vi "Sample_Panel_2.vi"(0 "HSMO#1":refnum<class "Hyper_State_Machine.lvclass">, 1 "State_Interval_Time(s)":dbl=0.025 min=0.0 max=86400.0 format="%#_13p", 2 "Time Target (s)":dbl=30.0 format="%#_13g", 3 "System_Delay(s)":dbl=0.05 min=0.0 max=86400.0 format="%#_13p") -> (8 "error out":errorcluster)   [LabVIEW 2021]
uses:
  C:/Program Files (x86)/Hyper State Machine Framework/SSW_Hyper_State_Machine.lvlibp/State_Machine_Class/Main_State_Machine/Hyper_State_Machine.lvclass
  C:/Program Files (x86)/Hyper State Machine Framework/SSW_Hyper_State_Machine.lvlibp/State_Machine_Class/State_Machine_Module.llb/State Machine.ctl
  C:/Program Files (x86)/Hyper State Machine Framework/SSW_Hyper_State_Machine.lvlibp/State_Machine_Class/State_Machine_Module.llb/State Machine[].ctl
  C:/Program Files (x86)/Hyper State Machine Framework/SSW_Hyper_State_Machine.lvlibp/State_Machine_Class/State_Machine_Module.llb/Iterval.ctl
  C:/Program Files (x86)/Hyper State Machine Framework/SSW_Hyper_State_Machine.lvlibp/State_Machine_Class/State_Machine_Module.llb/Lock_Unlock.ctl
  C:/Program Files (x86)/Hyper State Machine Framework/SSW_Hyper_State_Machine.lvlibp
panel:
  out "Running Mode":string
  out "This_State_Id":u32 format="%08x"
  out "Message from Child":string
  in  "Block Chain":bool=TRUE caption="Checkbox"
  in  "Message to Parent":string="I'm Child State"
  in  "Send":bool
  out "Parent_State_Id":u32 format="%08x"
  out "Panel_Close":bool=TRUE
  out "Active":bool=TRUE
  out "Implementation Class":string
  out "Current State":string
  out "Heartbeat":bool=TRUE
  in  "Unlock":bool
  in  "Reset":bool
  in  "lock All":bool
  in  "New_Windows":bool
  out "Timing":dbl
  out "Lock":bool
  # "HSMO#2"
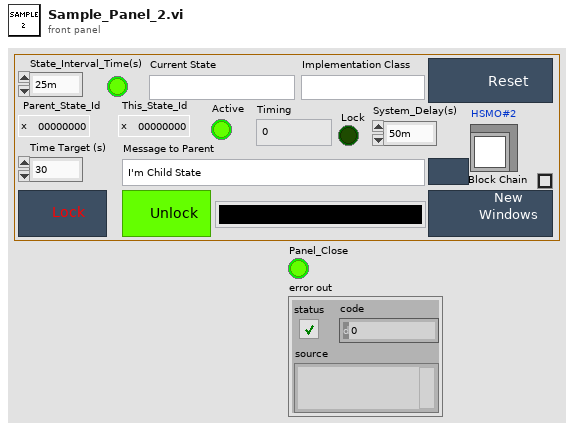
[diagram p1: front panel]
types:
  T1 = typedef "SSW_Hyper_State_Machine.lvlibp/State Machine.ctl" = cluster{"Command":string, "Data":variant}
  T2 = typedef "SSW_Hyper_State_Machine.lvlibp/Lock_Unlock.ctl" = cluster{"Action_Mode (Get)":enum16{"Set", "Get"}, "Action_Set (False)":bool, "State_In (Wait)":string}
  T3 = typedef "SSW_Hyper_State_Machine.lvlibp/State Machine[].ctl" = cluster{"Command":string, "Data":variant}[]
  T4 = typedef "SSW_Hyper_State_Machine.lvlibp/Iterval.ctl" = cluster{"Delay(s)":dbl, "State (Interval_Delay)":string}
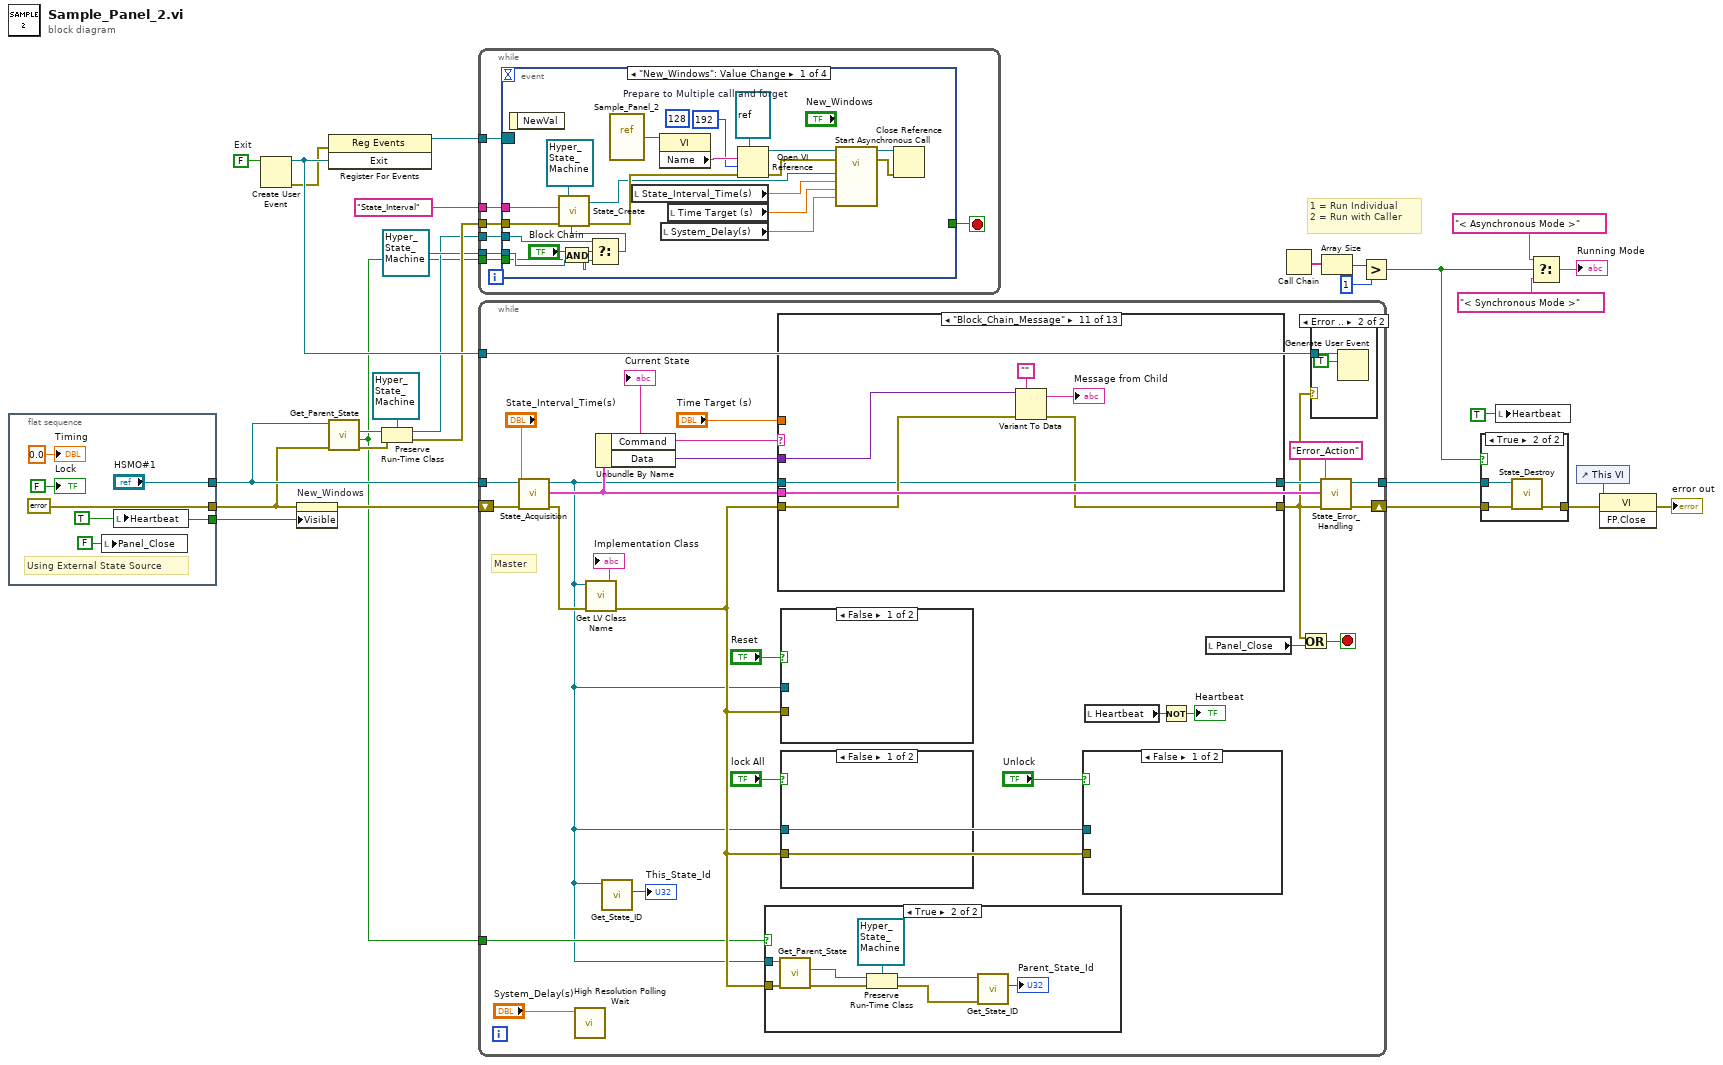
[diagram p0: block diagram]
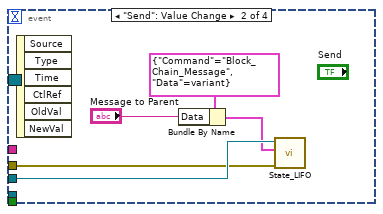
[diagram p3: hidden frame]
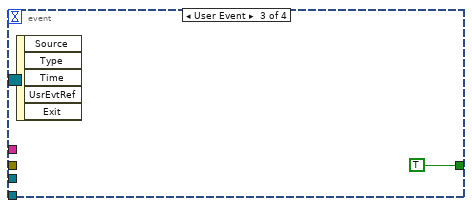
[diagram p4: hidden frame]
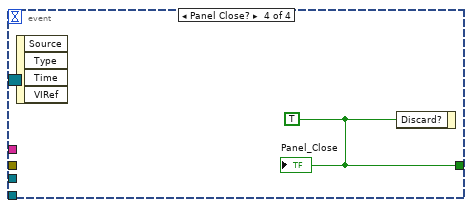
[diagram p5: hidden frame]
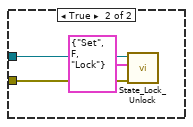
[diagram p8: hidden frame]
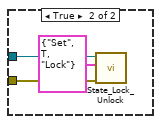
[diagram p9: hidden frame]
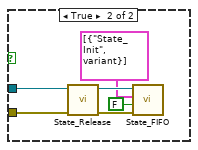
[diagram p10: hidden frame]
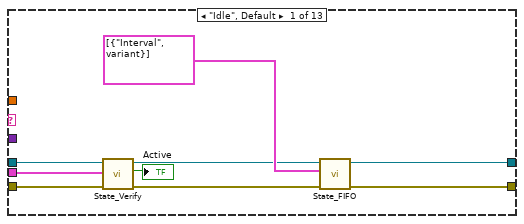
[diagram p11: hidden frame]
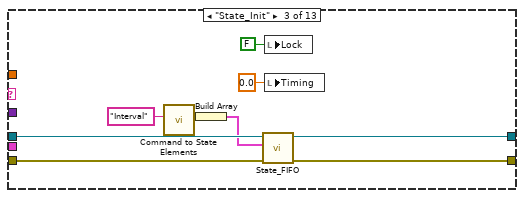
[diagram p13: hidden frame]
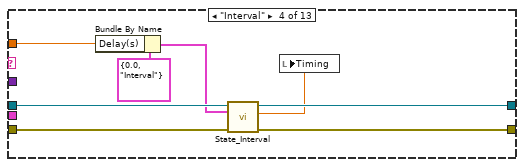
[diagram p14: hidden frame]
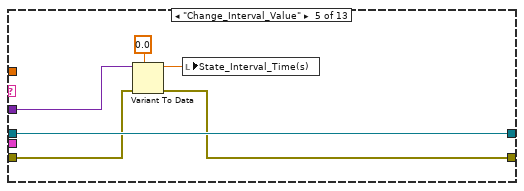
[diagram p15: hidden frame]
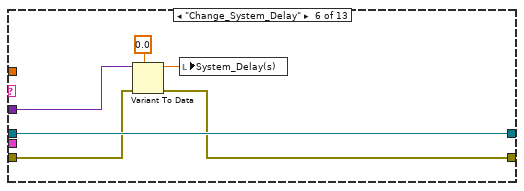
[diagram p16: hidden frame]
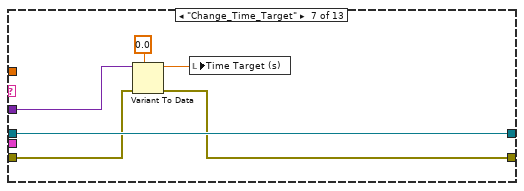
[diagram p17: hidden frame]
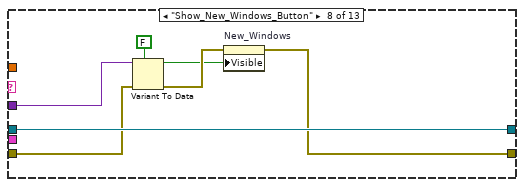
[diagram p18: hidden frame]
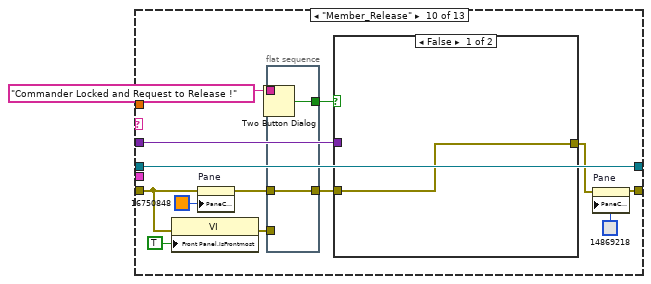
[diagram p20: hidden frame]
diagram:
  w26 = FALSE  # Exit
  # "1 = Run Individual\n2 = Run with Caller"
  n1 = flat-sequence {
    tunnel: ["HSMO#1"] -> w12
    tunnel: [errorcluster {"status"=FALSE, "code"=0, "source"=""} ("error out")] -> w11
    tunnel: [w31] -> w27
    frame #0 {
      w31 = TRUE ("Heartbeat")
      # "Using External State Source"
      n2 = local write "Panel_Close"(FALSE ("Panel_Close")) -> ()
      n3 = local write "Heartbeat"(w31) -> ()
      "Lock" <- FALSE ("Lock")
      "Timing" <- 0.0 ("Timing")
    }
  }
  n4 = Create User Event(user event datatype=w26) -> (user event=w24:refnum<user-event>, error out=w18:errorcluster)  [unwired: 1 in]
  n5 = property on="New_Windows" class="Bool"(error in=w11, "Visible"=w27) -> (error out=w28:errorcluster)  [unwired: 1 in, 1 out]
  n6 = register-events(error in=w18, w24) -> (reference out=w25:refnum<event-registration>)  [unwired: 1 in, 1 out]
  n7 = call-dynamic "Get_Parent_State.vi"("error in (no error)"=w11, "Hyper_State_Machine in"=w12) -> ("error out"=w10:errorcluster, "Paent_State_Status"=w9:bool, "Paent_State"=w13:refnum<class "State_Interface.lvclass">)  [unwired: 6 in, 1 out]
  n8 = Preserve Run-Time Class(object in=w13, error in=w10, 2:refnum<class "Hyper_State_Machine.lvclass"> refnum ("HSMO#1")) -> (object out=w14:refnum<class "Hyper_State_Machine.lvclass">, error out=w16:errorcluster)
  n9 = while {
    tunnel: w25 -> [w41]
    tunnel: "State_Interval" ("State_Interval_Name") -> [w40]
    tunnel: w16 -> [w39]
    tunnel: w14 -> [w38]
    tunnel: refnum<class "Hyper_State_Machine.lvclass"> refnum ("f") -> [w37]
    tunnel: w9 -> [w36]
    stop <- w42 stop-if-true
    n10 = event shown="[0] \"New_Windows\": Value Change" {
      selector: w41 -> [_ _ _ _]
      dyn-events: _ -> [_ _ _ _]
      timeout: _ -> [_ _ _ _]
      tunnel: [_ _ TRUE w71] -> w42
      tunnel: w40 -> [w52 _ _ _]
      tunnel: w39 -> [w51 w68 _ _]
      tunnel: w38 -> [w49 w69 _ _]
      tunnel: w37 -> [w48 _ _ _]
      tunnel: w36 -> [w44 _ _ _]
      event "New_Windows": Value Change {
        (unwired) 128 ("options")
        w43 = 192  # Prepare to Multiple call and forget
        n11 = event-data() -> ()  [unwired: 1 in, 1 out]
        n12 = And(x="Block Chain", y=w44) -> (x .and. y?=w45:bool)
        n13 = Select(t=w49, s=w45, f=w48) -> (s? t:f=w46:refnum<class "Hyper_State_Machine.lvclass">)
        n14 = call-dynamic "State_Create.vi"("Parent_State"=w46, "error in (no error)"=w51, "State_Interval_Name"=w52, "State_Machine_Class in"=refnum<class "Hyper_State_Machine.lvclass"> refnum) -> ("error out"=w53:errorcluster, "State_Machine_Class out"=w50:refnum<class "Hyper_State_Machine.lvclass">)  [unwired: 5 in, 1 out]
        n15 = vi-ref "Sample_Panel_2.vi"() -> (w64:refnum<vi>)
        n16 = local read "State_Interval_Time(s)"() -> (w57:dbl)
        n17 = property class="VI"(reference=w64) -> ("Name"=w63:string)  [unwired: 1 in, 2 out]
        n18 = local read "System_Delay(s)"() -> (w55:dbl)
        n19 = local read "Time Target (s)"() -> (w56:dbl)
        n20 = Open VI Reference(type specifier VI Refnum (for type only)=refnum<vi> refnum, vi path=w63, options=w43, error in (no error)=w53) -> (vi reference=w61:refnum<vi>, error out=w60:errorcluster)  [unwired: 2 in]
        n21 = call-by-ref "Start Asynchronous Call"(reference=w61, error in=w60, "HSMO#1"=w50, "State_Interval_Time(s)"=w57, "Time Target (s)"=w56, "System_Delay(s)"=w55) -> (reference out=w59:refnum<vi>, error out=w58:errorcluster)  [unwired: 4 in, 1 out]
        n22 = Close Reference(reference=w59, error in (no error)=w58) -> ()  [unwired: 1 out]
      }
      event "Send": Value Change {
        n23 = event-data() -> ()  [unwired: 1 in, 6 out]
        n24 = Bundle By Name(cluster=T1 {"Command"="Block_Chain_Message", "Data"=variant} ("State Machine"), "Data"="Message to Parent") -> (w65:T1)
        n25 = call-dynamic "State_LIFO.vi"("error in (no error)"=w68, "State Machine"=w65, "State_Machine_Class in"=w69) -> ()  [unwired: 7 in, 2 out]
      }
      event User Event {
        n26 = event-data() -> ()  [unwired: 1 in, 5 out]
      }
      event Panel Close? {
        w71 = TRUE ("Discard?")
        n27 = event-data() -> ()  [unwired: 1 in, 4 out]
        n28 = event-data("Discard?"=w71) -> ()  [unwired: 1 in, 1 out]
        "Panel_Close" <- w71
      }
    }
  }
  n29 = while {
    tunnel: w12 -> [w98]
    shift-right: [w80] -> w29
    shift-left: w28 -> [w97]
    tunnel: w24 -> [w81]
    tunnel: [w79] -> w20
    tunnel: w9 -> [w74]
    stop <- w76 stop-if-true
    # "Master"
    n30 = call-dynamic "State_Acquisition.vi"("error in (no error)"=w97, "State_Interval_Time(s)"="State_Interval_Time(s)", "Main_Machine_State_Class in"=w98) -> ("error out"=w84:errorcluster, "State"=w82:T1, "Main_Machine_State_Class out"=w72:refnum<class "Hyper_State_Machine.lvclass">)  [unwired: 2 in, 4 out]
    n31 = call <vilib>:"High Resolution Polling Wait.vi"("seconds to wait"="System_Delay(s)") -> ()  [unwired: 10 in, 1 out]
    n32 = call <vilib>:"Get LV Class Name.vi"("error in (no error)"=w84, "object"=w72) -> ("error out"=w75:errorcluster, "class name"=→"Implementation Class":string)  [unwired: 8 in]
    n33 = Unbundle By Name(w82) -> ("Command"=w86:string, "Data"=w89:variant)
    "Current State" <- w86
    n34 = call-dynamic "Get_State_ID.vi"("Hyper_State_Machine in"=w72) -> ("State_ID"=→"This_State_Id":u32)  [unwired: 8 in, 2 out]
    n35 = case shown="True" w74 {
      tunnel: w72 -> [_ w102]
      tunnel: w75 -> [_ w101]
      frame False {
      }
      frame True {
        n36 = call-dynamic "Get_Parent_State.vi"("error in (no error)"=w101, "Hyper_State_Machine in"=w102) -> ("error out"=w99:errorcluster, "Paent_State"=w100:refnum<class "State_Interface.lvclass">)  [unwired: 6 in, 2 out]
        n37 = Preserve Run-Time Class(object in=w100, error in=w99, 2:refnum<class "Hyper_State_Machine.lvclass"> refnum ("HSMO#1")) -> (object out=w104:refnum<class "Hyper_State_Machine.lvclass">, error out=w103:errorcluster)
        n38 = call-dynamic "Get_State_ID.vi"("error in (no error)"=w103, "Hyper_State_Machine in"=w104) -> ("State_ID"=→"Parent_State_Id":u32)  [unwired: 7 in, 2 out]
      }
    }
    n39 = case shown="\"Block_Chain_Message\"" w86 {
      tunnel: w89 -> [_ _ _ _ w153 w159 w165 w172 _ w187 w204 _ _]
      tunnel: w72 -> [w126 w131 w140 w146 w154 w160 w166 w173 w175 w188 w202 w211 w218]
      tunnel: w75 -> [w125 w130 w138 w145 w152 w158 w164 w171 w174 w182 w203 w210 w217]
      tunnel: [w129 w131 w139 w143 w154 w160 w166 w173 w175 w188 w202 w209 w216] -> w87
      tunnel: [w128 w130 w137 w142 w151 w157 w163 w167 w174 w177 w201 w208 w212] -> w77
      tunnel: "Time Target (s)" -> [_ _ _ w148 _ _ _ _ _ _ _ _ _]
      tunnel: w82 -> [w124 _ _ _ _ _ _ _ _ _ _ _ _]
      frame "Idle", Default {
        n40 = call-dynamic "State_Verify.vi"("error in (no error)"=w125, "State(Idle)"=w124, "State_Machine_Class in"=w126) -> ("error out"=w122:errorcluster, "Active"=→"Active":bool, "State_Machine_Class out"=w123:refnum<class "Hyper_State_Machine.lvclass">)  [unwired: 6 in]
        n41 = call-dynamic "State_FIFO.vi"("error in (no error)"=w122, "State Machine[]"=T3 [{"Command"="Interval", "Data"=variant}], "State_Machine_Class in"=w123) -> ("error out"=w128:errorcluster, "State_Machine_Class out"=w129:refnum<class "Hyper_State_Machine.lvclass">)  [unwired: 7 in]
      }
      frame "State_Interval" {
        # "Execute Every Define of State Interval Time"
      }
      frame "State_Init" {
        n42 = call "Command to State Elements.vi"("Command"="Interval") -> ("Command to State Elements"=w135:T1)  [unwired: 10 in]
        n43 = Build Array(w135) -> (w134:T1[])
        n44 = call-dynamic "State_FIFO.vi"("error in (no error)"=w138, "State Machine[]"=w134, "State_Machine_Class in"=w140) -> ("error out"=w137:errorcluster, "State_Machine_Class out"=w139:refnum<class "Hyper_State_Machine.lvclass">)  [unwired: 7 in]
        n45 = local write "Lock"(FALSE ("Lock")) -> ()
        n46 = local write "Timing"(0.0 ("Timing")) -> ()
      }
      frame "Interval" {
        n47 = Bundle By Name(cluster=T4 {"Delay(s)"=0.0, "State (Interval_Delay)"="Interval"} ("Parameter"), "Delay(s)"=w148) -> (w144:T4)
        n48 = call-dynamic "State_Interval.vi"("error in (no error)"=w145, "Parameter"=w144, "State_Machine_Class in"=w146) -> ("error out"=w142:errorcluster, "Elapsed Time(s)"=w141:dbl, "State_Machine_Class out"=w143:refnum<class "Hyper_State_Machine.lvclass">)  [unwired: 6 in]
        n49 = local write "Timing"(w141) -> ()
      }
      frame "Change_Interval_Value" {
        n50 = Variant To Data(error in=w152, type=0.0 ("Time Target (s)"), Variant=w153) -> (data=w149:dbl, error out=w151:errorcluster)
        n51 = local write "State_Interval_Time(s)"(w149) -> ()
      }
      frame "Change_System_Delay" {
        n52 = Variant To Data(error in=w158, type=0.0 ("Time Target (s)"), Variant=w159) -> (data=w155:dbl, error out=w157:errorcluster)
        n53 = local write "System_Delay(s)"(w155) -> ()
      }
      frame "Change_Time_Target" {
        n54 = Variant To Data(error in=w164, type=0.0 ("Time Target (s)"), Variant=w165) -> (data=w161:dbl, error out=w163:errorcluster)
        n55 = local write "Time Target (s)"(w161) -> ()
      }
      frame "Show_New_Windows_Button" {
        n56 = Variant To Data(error in=w171, type=FALSE, Variant=w172) -> (data=w168:bool, error out=w169:errorcluster)
        n57 = property on="New_Windows" class="Bool"(error in=w169, "Visible"=w168) -> (error out=w167:errorcluster)  [unwired: 1 in, 1 out]
      }
      frame "Error_Action" {
      }
      frame "Member_Release" {
        n58 = property class="VI"(error in=w182, "Front Panel.IsFrontmost"=TRUE ("Front Panel Window:Is Frontmost")) -> (error out=w176:errorcluster)  [unwired: 1 in, 1 out]
        n59 = property on="Pane" class="Pane"(error in=w182, "PaneColor"=u32 16750848 ("Pane Color")) -> (error out=w181:errorcluster)  [unwired: 1 in, 1 out]
        n60 = flat-sequence {
          tunnel: "Commander Locked and Request to Release !" ("message") -> [w191]
          tunnel: [w190] -> w185
          tunnel: [w189] -> w180
          tunnel: w181 -> [w189]
          tunnel: w176 -> [_]
          frame #0 {
            n61 = Two Button Dialog(message=w191) -> (T button?=w190:bool)  [unwired: 2 in]
          }
        }
        n62 = case shown="False" w185 {
          tunnel: w180 -> [w192 w199]
          tunnel: w187 -> [_ w198]
          tunnel: [w192 w197] -> w178
          frame False {
          }
          frame True {
            n63 = Variant To Data(error in=w199, type=refnum<class "Hyper_State_Machine.lvclass"> refnum ("HSMO#1"), Variant=w198) -> (data=w195:refnum<class "Hyper_State_Machine.lvclass">, error out=w194:errorcluster)
            n64 = call-dynamic "State_Lock_Unlock.vi"("error in (no error)"=w194, "Parameter"=T2 {"Action_Mode (Get)"=enum."Set", "Action_Set (False)"=FALSE, "State_In (Wait)"="Lock"}, "State_Machine_Class in"=w195) -> ("error out"=w197:errorcluster)  [unwired: 6 in, 2 out]
          }
        }
        n65 = property on="Pane" class="Pane"(error in=w178, "PaneColor"=u32 14869218 ("Pane Color")) -> (error out=w177:errorcluster)  [unwired: 1 in, 1 out]
      }
      frame "Block_Chain_Message" {
        n66 = Variant To Data(error in=w203, type="", Variant=w204) -> (data=→"Message from Child":string, error out=w201:errorcluster)
      }
      frame "Lock" {
        n67 = call-dynamic "State_Lock_Unlock.vi"("error in (no error)"=w210, "Parameter"=T2 {"Action_Mode (Get)"=enum."Get", "Action_Set (False)"=FALSE, "State_In (Wait)"="Lock"}, "State_Machine_Class in"=w211) -> ("error out"=w208:errorcluster, "Action_Get"=w206:bool, "State_Machine_Class out"=w209:refnum<class "Hyper_State_Machine.lvclass">)  [unwired: 6 in]
        n68 = local write "Lock"(w206) -> ()
      }
      frame "Exit" {
        n69 = call-dynamic "State_Release.vi"("error in (no error)"=w217, "State_Machine_Class in"=w218) -> ("error out"=w214:errorcluster, "State_Machine_Class out"=w215:refnum<class "Hyper_State_Machine.lvclass">)  [unwired: 8 in]
        n70 = call-dynamic "State_Lock_Unlock.vi"("error in (no error)"=w214, "Parameter"=T2 {"Action_Mode (Get)"=enum."Set", "Action_Set (False)"=FALSE, "State_In (Wait)"="Lock"}, "State_Machine_Class in"=w215) -> ("error out"=w212:errorcluster, "State_Machine_Class out"=w216:refnum<class "Hyper_State_Machine.lvclass">)  [unwired: 6 in, 1 out]
      }
    }
    n71 = case shown="False" "Reset" {
      tunnel: w72 -> [_ w120]
      tunnel: w75 -> [_ w116]
      frame False {
      }
      frame True {
        n72 = call-dynamic "State_Release.vi"("error in (no error)"=w116, "State_Machine_Class in"=w120) -> ("error out"=w118:errorcluster, "State_Machine_Class out"=w119:refnum<class "Hyper_State_Machine.lvclass">)  [unwired: 8 in]
        n73 = call-dynamic "State_FIFO.vi"("error in (no error)"=w118, "State_Interval(Enable)"=FALSE, "State Machine[]"=T3 [{"Command"="State_Init", "Data"=variant}], "State_Machine_Class in"=w119) -> ()  [unwired: 6 in, 2 out]
      }
    }
    n74 = case shown="False" "lock All" {
      tunnel: w72 -> [_ w114]
      tunnel: w75 -> [_ w113]
      frame False {
      }
      frame True {
        n75 = call-dynamic "State_Lock_Unlock.vi"("error in (no error)"=w113, "Parameter"=T2 {"Action_Mode (Get)"=enum."Set", "Action_Set (False)"=TRUE, "State_In (Wait)"="Lock"}, "State_Machine_Class in"=w114) -> ()  [unwired: 6 in, 3 out]
      }
    }
    n76 = case shown="False" "Unlock" {
      tunnel: w72 -> [_ w110]
      tunnel: w75 -> [_ w111]
      frame False {
      }
      frame True {
        n77 = call-dynamic "State_Lock_Unlock.vi"("error in (no error)"=w111, "Parameter"=T2 {"Action_Mode (Get)"=enum."Set", "Action_Set (False)"=FALSE, "State_In (Wait)"="Lock"}, "State_Machine_Class in"=w110) -> ()  [unwired: 6 in, 3 out]
      }
    }
    n78 = local read "Heartbeat"() -> (w91:bool)
    n79 = Not(x=w91) -> (.not. x?=→"Heartbeat":bool)
    n80 = local read "Panel_Close"() -> (w78:bool)
    n81 = Or(x=w77, y=w78) -> (x .or. y?=w76:bool)
    n82 = case shown="Error .." w77 {
      tunnel: w81 -> [_ w107]
      frame No Error {
      }
      frame Error {
        n83 = Generate User Event(user event=w107, event data cluster=TRUE ("event data")) -> ()  [unwired: 2 in, 2 out]
      }
    }
    n84 = call-dynamic "State_Error_Handling.vi"("error in (no error)"=w77, "Reply_State_Name"="Error_Action", "Handling_State(State_Acquisition)"=w82, "State_Machine_Class in"=w87) -> ("error out"=w80:errorcluster, "State_Machine_Class out"=w79:refnum<class "Hyper_State_Machine.lvclass">)  [unwired: 6 in]
  }
  n85 = Call Chain() -> (call chain=w23:string[])
  n86 = Array Size(array=w23) -> (size(s)=w22:i32)
  n87 = Greater?(x=w22, y=1) -> (0:w1:bool)
  n88 = case shown="True" w1 {
    tunnel: w29 -> [w219 w222]
    tunnel: w20 -> [_ w221]
    tunnel: [w219 w220] -> w6
    frame False {
    }
    frame True {
      n89 = call-dynamic "State_Destroy.vi"("error in (no error)"=w222, "State_Machine_Class in"=w221) -> ("error out"=w220:errorcluster)  [unwired: 9 in]
    }
  }
  n90 = local write "Heartbeat"(TRUE ("Show_Stop_Button")) -> ()
  n91 = Select(t="< Asynchronous Mode >", s=w1, f="< Synchronous Mode >") -> (s? t:f=→"Running Mode":string)
  n92 = control-ref of="This VI"() -> (w7:refnum<vi>)
  n93 = invoke class="VI" method="FP.Close"(reference=w7, error in=w6) -> (error out=→"error out":errorcluster)  [unwired: 1 in, 2 out]
